vi "CMN_SendAsyncMsg_dhe.vi"(7 "type":enum16{"ERROR", "WARNING", "INFO", "CHANGED"}(ring)=enum."INFO", 9 "Message":string, 10 "device":string, 11 "command":string) -> ()   [LabVIEW 2016]
uses:
  DBSHAND/private/vis/DatabaseHand_Element_Get(string).vi
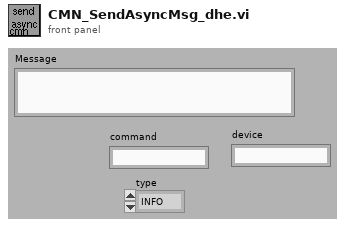
[diagram p1: front panel]
types:
  T1 = typedef "DatabaseHand_RefNum.ctl" = refnum<vi>
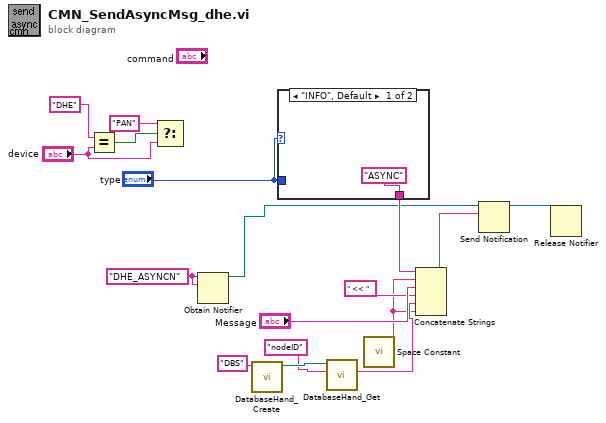
[diagram p0: block diagram]
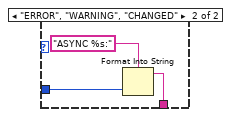
[diagram p2: hidden frame]
diagram:
  w10 = "DHE_ASYNCN" ("name (unnamed)")
  n1 = Equal?(x="DHE" ("y"), y="device") -> (x = y?=w17:bool)
  n2 = Select(t="PAN", s=w17, f="device") -> ()  [unwired: 1 out]
  n3 = Obtain Notifier(name (unnamed)=w10, notification data type=w10) -> (notifier out=w9:refnum<notifier>)  [unwired: 2 in, 2 out]
  n4 = call "DatabaseHand_Create.vi"("Name"="DBS") -> ("Database RefNum out"=w5:T1)  [unwired: 1 in, 9 out]
  n5 = case shown="\"INFO\", Default" "type" {
    tunnel: "type" -> [_ w21]
    tunnel: ["ASYNC" w19] -> w12
    frame "INFO", Default {
    }
    frame "ERROR", "WARNING", "CHANGED" {
      n6 = Format Into String(format string="ASYNC %s:", w21) -> (resulting string=w19:string)  [unwired: 2 in, 1 out]
    }
  }
  n7 = call-poly "DatabaseHand_Get.vi"("name"="nodeID", "Database RefNum in"=w5) -> ("value"=w2:string)  [unwired: 3 in, 6 out]
  n8 = call <vilib>:"Space Constant.vi"() -> ("String"=w1:string)
  n9 = Concatenate Strings(w12, w1, "Message", " << " ("string"), w2, w1) -> (w13:string)
  n10 = Send Notification(notification=w13, notifier=w9) -> (notifier out=w11:refnum<notifier>)  [unwired: 1 in, 1 out]
  n11 = Release Notifier(notifier=w11) -> ()  [unwired: 1 in, 4 out]
